vi "Diffusivity 32f.vi"(8 "Error In":errorcluster, 11 "Anisotropic Filter Object":T1={"Device In"=0, "Convolution Object"={"Device In"=0, "Program Handle"=0, "Kernel Memory Object"={"Device ID"=0, "Memeroy ID"=0, "Dimension"={"Depth"=0, "Height"=0, "Width"=0}, "Memory Type"=enum."32f"}, "Convolved Memory Object"={"Device ID"=0, "Memeroy ID"=0, "Dimension"={"Depth"=0, "Height"=0, "Width"=0}, "Memory Type"=enum."32f"}}, "Imag Kernel"=[], "Real Kernel"=[], "Convolved Buffer"={"Device ID"=0, "Memeroy ID"=0, "Dimension"={"Depth"=0, "Height"=0, "Width"=0}, "Memory Type"=enum."32f"}, "Program Handle"=0, "Ansiotropic Filter Parameters"={"Time Step"=0.0, "Total Time"=0.5, "Std. Deviation"=0.0, "Gaussian Filter X Size"=1, "Gaussian Filter Y Size"=1, "Gaussian Filter Z Size"=1}, "Raw Data"={"Device ID"=0, "Memeroy ID"=0, "Dimension"={"Depth"=0, "Height"=0, "Width"=0}, "Memory Type"=enum."32f"}, "Buffer 3"={"Device ID"=0, "Memeroy ID"=0, "Dimension"={"Depth"=0, "Height"=0, "Width"=0}, "Memory Type"=enum."32f"}, "Dimensions"={"Depth"=1, "Height"=1, "Width"=1}} {"Dimensions"."Width" min=1; "Dimensions"."Height" min=1; "Dimensions"."Depth" min=1; "Buffer 3"."Dimension"."Width" min=1; "Buffer 3"."Dimension"."Height" min=1; "Buffer 3"."Dimension"."Depth" min=1; "Raw Data"."Dimension"."Width" min=1; "Raw Data"."Dimension"."Height" min=1; "Raw Data"."Dimension"."Depth" min=1; "Ansiotropic Filter Parameters"."Gaussian Filter Z Size" min=1 max=99 step=2; "Ansiotropic Filter Parameters"."Gaussian Filter Y Size" min=1 max=99 step=2; "Ansiotropic Filter Parameters"."Gaussian Filter X Size" min=1 max=99 step=2; "Convolved Buffer"."Dimension"."Width" min=1; "Convolved Buffer"."Dimension"."Height" min=1; "Convolved Buffer"."Dimension"."Depth" min=1; "Convolution Object"."Convolved Memory Object"."Dimension"."Width" min=1; "Convolution Object"."Convolved Memory Object"."Dimension"."Height" min=1; "Convolution Object"."Convolved Memory Object"."Dimension"."Depth" min=1; "Convolution Object"."Kernel Memory Object"."Dimension"."Width" min=1; "Convolution Object"."Kernel Memory Object"."Dimension"."Height" min=1; "Convolution Object"."Kernel Memory Object"."Dimension"."Depth" min=1}) -> (0 "Error Out":errorcluster, 3 "Anisotropic Filter Object Out":T1={"Device In"=0, "Convolution Object"={"Device In"=0, "Program Handle"=0, "Kernel Memory Object"={"Device ID"=0, "Memeroy ID"=0, "Dimension"={"Depth"=0, "Height"=0, "Width"=0}, "Memory Type"=enum."32f"}, "Convolved Memory Object"={"Device ID"=0, "Memeroy ID"=0, "Dimension"={"Depth"=0, "Height"=0, "Width"=0}, "Memory Type"=enum."32f"}}, "Imag Kernel"=[], "Real Kernel"=[], "Convolved Buffer"={"Device ID"=0, "Memeroy ID"=0, "Dimension"={"Depth"=0, "Height"=0, "Width"=0}, "Memory Type"=enum."32f"}, "Program Handle"=0, "Ansiotropic Filter Parameters"={"Time Step"=0.0, "Total Time"=0.5, "Std. Deviation"=0.0, "Gaussian Filter X Size"=1, "Gaussian Filter Y Size"=1, "Gaussian Filter Z Size"=1}, "Raw Data"={"Device ID"=0, "Memeroy ID"=0, "Dimension"={"Depth"=0, "Height"=0, "Width"=0}, "Memory Type"=enum."32f"}, "Buffer 3"={"Device ID"=0, "Memeroy ID"=0, "Dimension"={"Depth"=0, "Height"=0, "Width"=0}, "Memory Type"=enum."32f"}, "Dimensions"={"Depth"=1, "Height"=1, "Width"=1}} {"Dimensions"."Width" min=1; "Dimensions"."Height" min=1; "Dimensions"."Depth" min=1; "Buffer 3"."Dimension"."Width" min=1; "Buffer 3"."Dimension"."Height" min=1; "Buffer 3"."Dimension"."Depth" min=1; "Raw Data"."Dimension"."Width" min=1; "Raw Data"."Dimension"."Height" min=1; "Raw Data"."Dimension"."Depth" min=1; "Ansiotropic Filter Parameters"."Gaussian Filter Z Size" min=1 max=99 step=2; "Ansiotropic Filter Parameters"."Gaussian Filter Y Size" min=1 max=99 step=2; "Ansiotropic Filter Parameters"."Gaussian Filter X Size" min=1 max=99 step=2; "Convolved Buffer"."Dimension"."Width" min=1; "Convolved Buffer"."Dimension"."Height" min=1; "Convolved Buffer"."Dimension"."Depth" min=1; "Convolution Object"."Convolved Memory Object"."Dimension"."Width" min=1; "Convolution Object"."Convolved Memory Object"."Dimension"."Height" min=1; "Convolution Object"."Convolved Memory Object"."Dimension"."Depth" min=1; "Convolution Object"."Kernel Memory Object"."Dimension"."Width" min=1; "Convolution Object"."Kernel Memory Object"."Dimension"."Height" min=1; "Convolution Object"."Kernel Memory Object"."Dimension"."Depth" min=1}, 4 "Time in ms":dbl)   [LabVIEW 2012, in "OpenCLV x64.lvlib"]
uses:
  OpenCLV x64.lvlib
  Controls/Anisotropic Filter Object.ctl
  Controls/Device ID.ctl
  Controls/Convolution Object.ctl
  Controls/Program Handle.ctl
  Controls/Memory Object.ctl
  Controls/Memory ID.ctl
  User Controls/Array Dimensions.ctl
  Controls/Memory Type.ctl
  Controls/Anisotropic Filter Parameters.ctl
  Set Kernel Arguments/Set Kernel Arguments Memory Object.vi
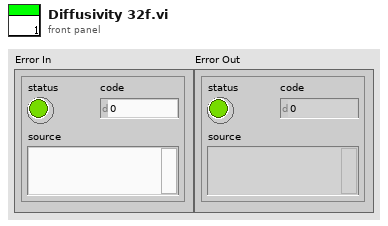
[diagram p1: front panel]
types:
  T1 = typedef "OpenCLV x64.lvlib/Anisotropic Filter Object.ctl" = cluster{"Device In":T2, "Convolution Object":T3, "Imag Kernel":sgl[][][], "Real Kernel":sgl[][][], "Convolved Buffer":T5, "Program Handle":T4, "Ansiotropic Filter Parameters":T9, "Raw Data":T5, "Buffer 3":T5, "Dimensions":T7}
  T2 = typedef "OpenCLV x64.lvlib/Device ID.ctl" = u64
  T3 = typedef "OpenCLV x64.lvlib/Convolution Object.ctl" = cluster{"Device In":T2, "Program Handle":T4, "Kernel Memory Object":T5, "Convolved Memory Object":T5}
  T4 = typedef "OpenCLV x64.lvlib/Program Handle.ctl" = u64
  T5 = typedef "OpenCLV x64.lvlib/Memory Object.ctl" = cluster{"Device ID":T2, "Memeroy ID":T6, "Dimension":T7, "Memory Type":T8}
  T6 = typedef "OpenCLV x64.lvlib/Memory ID.ctl" = u64
  T7 = typedef "Array Dimensions.ctl" = cluster{"Depth":u64, "Height":u64, "Width":u64}
  T8 = typedef "OpenCLV x64.lvlib/Memory Type.ctl" = enum16{"32f", "u8", "i8", "u16", "i16", "u32", "i32", "64f"}
  T9 = typedef "OpenCLV x64.lvlib/Anisotropic Filter Parameters.ctl" = cluster{"Time Step":sgl, "Total Time":sgl, "Std. Deviation":sgl, "Gaussian Filter X Size":u32, "Gaussian Filter Y Size":u32, "Gaussian Filter Z Size":u32}
  T10 = typedef "OpenCLV x64.lvlib/Kernel Handle.ctl" = u64
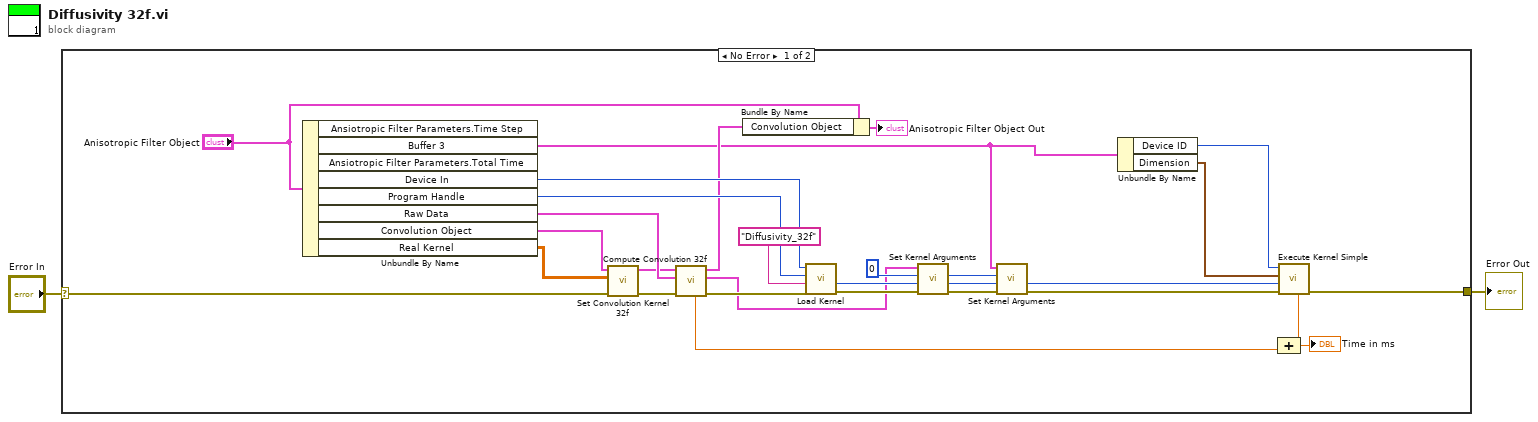
[diagram p0: block diagram]
diagram:
  n1 = case shown="No Error" "Error In" {
    selector: "Error In" -> [w31 w32]
    tunnel: [w17 w32] -> w1
    frame No Error {
      n2 = Unbundle By Name("Anisotropic Filter Object") -> ("Buffer 3"=w5:T5, "Device In"=w29:T2, "Program Handle"=w30:T4, "Raw Data"=w20:T5, "Convolution Object"=w22:T3, "Real Kernel"=w9:sgl[][][])  [unwired: 2 out]
      n3 = call "Set Convolution Kernel 32f.vi"("Error In"=w31, "Kernel In"=w9, "Convolution Object"=w22) -> ("Error Out"=w21:errorcluster, "Convolution Object Out"=w15:T3)  [unwired: 7 in]
      n4 = call "Compute Convolution 32f.vi"("Error In"=w21, "Input Memory"=w20, "Convolution Object"=w15) -> ("Error Out"=w19:errorcluster, "Convolved Memory"=w18:T5, "Convolution Object Out"=w11:T3, "Time in ms"=w24:dbl)  [unwired: 5 in]
      n5 = Bundle By Name(cluster="Anisotropic Filter Object", "Convolution Object"=w11) -> (→"Anisotropic Filter Object Out":T1)
      n6 = call "Load Kernel.vi"("Error In"=w19, "Kernel Name"="Diffusivity_32f", "Program Handle"=w30, "Device In"=w29) -> ("Error Out"=w27:errorcluster, "Kernel Handle"=w26:T10)  [unwired: 4 in, 2 out]
      n7 = call-poly "Set Kernel Arguments.vi"("Error In"=w27, "Kernel Handle"=w26, "Argument Number"=0, "Memory Object"=w18) -> ("Error Out"=w8:errorcluster, "Kernel Handle out"=w7:T10, "Auto Inc Arugment Number"=w6:i32)  [unwired: 5 in]
      n8 = call-poly "Set Kernel Arguments.vi"("Error In"=w8, "Kernel Handle"=w7, "Argument Number"=w6, "Memory Object"=w5) -> ("Error Out"=w4:errorcluster, "Kernel Handle out"=w3:T10)  [unwired: 5 in, 1 out]
      n9 = Unbundle By Name(w5) -> ("Device ID"=w14:T2, "Dimension"=w13:T7)
      n10 = call "Execute Kernel Simple.vi"("Error In"=w4, "Kernel Handle"=w3, "Thread Dimensions"=w13, "Device In"=w14) -> ("Error Out"=w17:errorcluster, "Time in ms"=w16:dbl)  [unwired: 4 in, 2 out]
      n11 = Compound Arithmetic op=ADD(w16, w24) -> (→"Time in ms":dbl)
    }
    frame Error {
    }
  }
  "Error Out" <- w1
